vi "Ini_Files.vi"() -> ()   [LabVIEW 2013]
panel:
  out "Paths ini files":T1
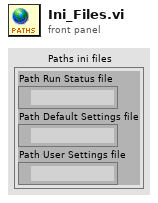
[diagram p1: front panel]
types:
  T1 = cluster{"Path Run Status file":path, "Path Default Settings file":path, "Path User Settings file":path}
diagram:
